vi "Process - Get Current.vi"(0 "Module Data In":T4, 11 "error in (no error)":errorcluster) -> (3 "|Current Process":T3, 4 "Module Data Out":T4, 6 "Process":T2, 8 "Status":T1, 10 "Data":variant, 15 "error out":errorcluster)   [LabVIEW 2017, in "Error Handler - Logger.lvlib"]
doc: "Get the current process that the Module must go through"
uses:
  Error Handler - Logger.lvlib
  Controls/Module - Data.ctl
  Modules.ctl
  Controls/Module - States.ctl
  Controls/Timing - Data.ctl
  Controls/Process - Element.ctl
  Controls/Process.ctl
  Controls/Process - Status.ctl
  Controls/Current Error Details.ctl
  Controls/Error Types.ctl
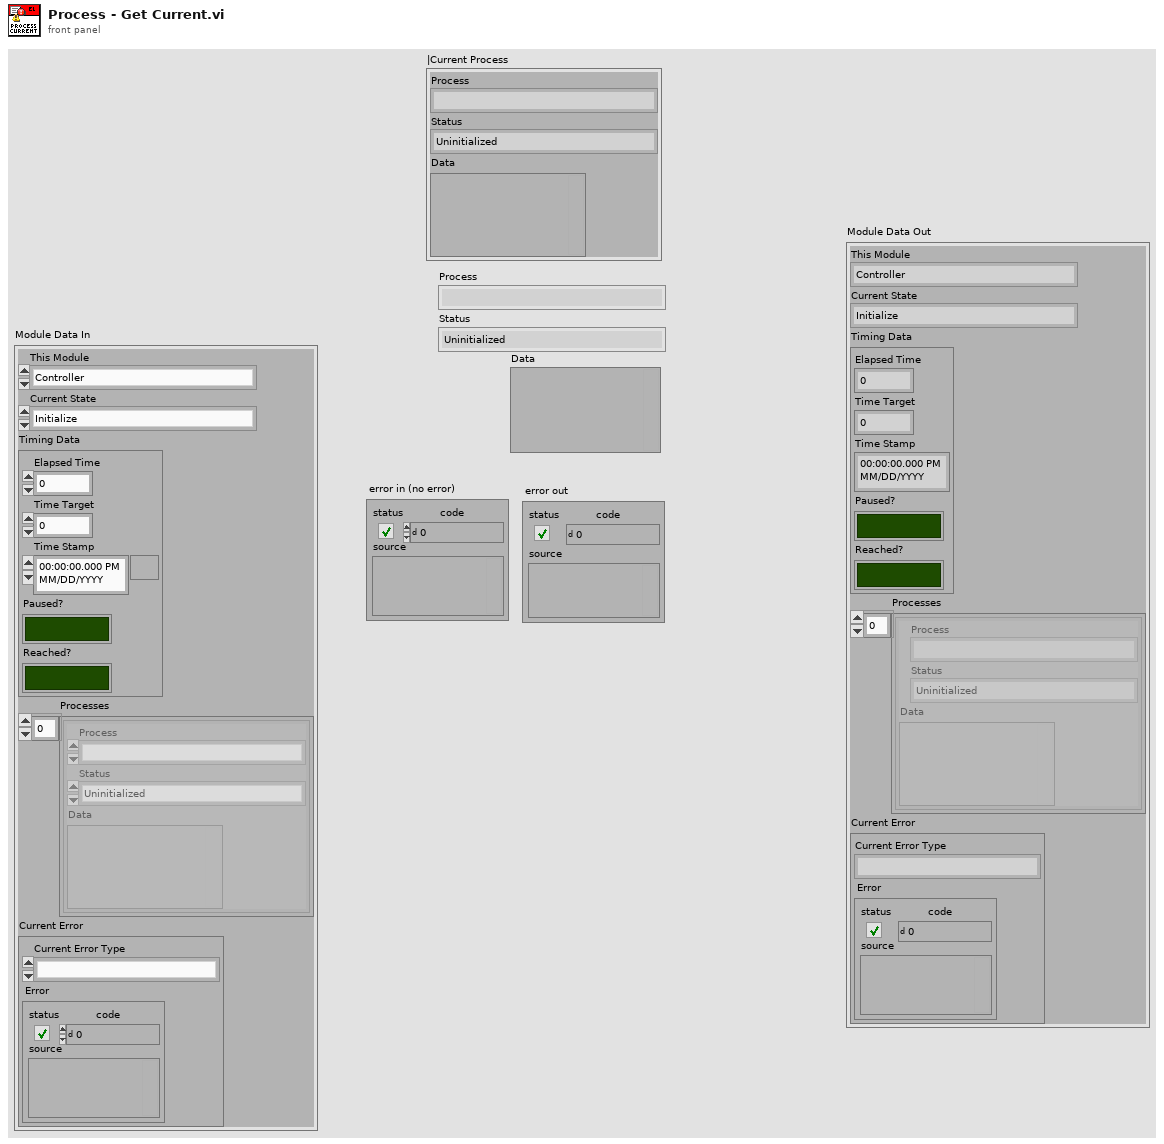
[diagram p1: front panel]
types:
  T1 = typedef "Error Handler - Logger.lvlib/Process - Status.ctl" = enum16{"Uninitialized", "Busy"}
  T2 = typedef "Error Handler - Logger.lvlib/Process.ctl" = enum16{""}
  T3 = typedef "Error Handler - Logger.lvlib/Process - Element.ctl" = cluster{"Process":T2, "Status":T1, "Data":variant}
  T4 = typedef "Error Handler - Logger.lvlib/Module - Data.ctl" = cluster{"This Module":T5, "Current State":T6, "Timing Data":T7, "Processes":T3[], "Current Error":T8}
  T5 = typedef "Error Handler - Logger.lvlib/Modules.ctl" = enum16{"Controller", "Error Handler - Logger"}
  T6 = typedef "Error Handler - Logger.lvlib/Module - States.ctl" = enum16{"Initialize", "Event ", "Send data", "FP Element: Update", "FP Element: Disable/Enable", "Timer: Setup", "Terminate", "--------Template----------", "Process Error", "Log ", "Log Error"}
  T7 = typedef "Error Handler - Logger.lvlib/Timing - Data.ctl" = cluster{"Elapsed Time":dbl, "Time Target":dbl, "Time Stamp":timestamp, "Paused?":bool, "Reached?":bool}
  T8 = typedef "Error Handler - Logger.lvlib/Current Error Details.ctl" = cluster{"Current Error Type":T9, "Error":errorcluster}
  T9 = typedef "Error Handler - Logger.lvlib/Error Types.ctl" = enum16{""}
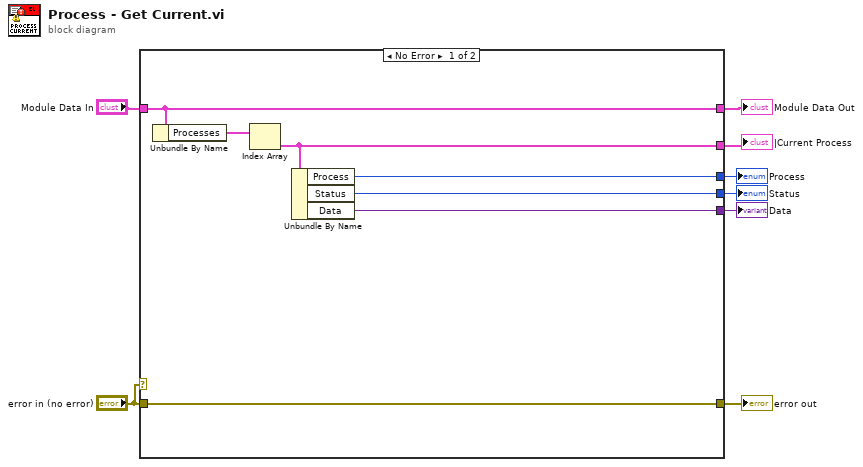
[diagram p0: block diagram]
diagram:
  n1 = case shown="No Error" "error in (no error)" {
    tunnel: [w14 w17] -> w8
    tunnel: "Module Data In" -> [w14 w17]
    tunnel: [w15 w16] -> w6
    tunnel: "error in (no error)" -> [w15 w16]
    tunnel: [w12 _] -> w4
    tunnel: [w11 _] -> w3
    tunnel: [w10 _] -> w2
    tunnel: [w9 _] -> w1
    frame No Error {
      n2 = Unbundle By Name(w14) -> ("Processes"=w13:T3[])
      n3 = Index Array(array=w13) -> (element=w9:T3)  [unwired: 1 in]
      n4 = Unbundle By Name(w9) -> ("Process"=w12:T2, "Status"=w11:T1, "Data"=w10:variant)
    }
    frame Error {
    }
  }
  "error out" <- w6
  "Module Data Out" <- w8
  "|Current Process" <- w1
  "Process" <- w4
  "Status" <- w3
  "Data" <- w2
